vi "View Data.vi"() -> ()   [LabVIEW 2019]
panel:
  in  "X":u16(ring) items=["F1:TIME", "F1:T-TYPE TC #1", "F1:", "F1:"]
  in  "Data File 4":path
  in  "Data File 3":path
  in  "Data File 2":path
  in  "Data File 1":path
  in  "Display Type":enum16{"Stacked Display", "Combined Display"}(ring)
  in  "Y4":u16(ring) items=["F1:TIME", "F1:T-TYPE TC #1", "F1:", "F1:"]
  in  "Y3":u16(ring) items=["F1:TIME", "F1:T-TYPE TC #1", "F1:", "F1:"]
  in  "Y2":u16(ring) items=["F1:TIME", "F1:T-TYPE TC #1", "F1:", "F1:"]
  in  "Y1":u16(ring) items=["F1:TIME", "F1:T-TYPE TC #1", "F1:", "F1:"]
  out "Graph":cluster{dbl[], dbl[]}[](graph)
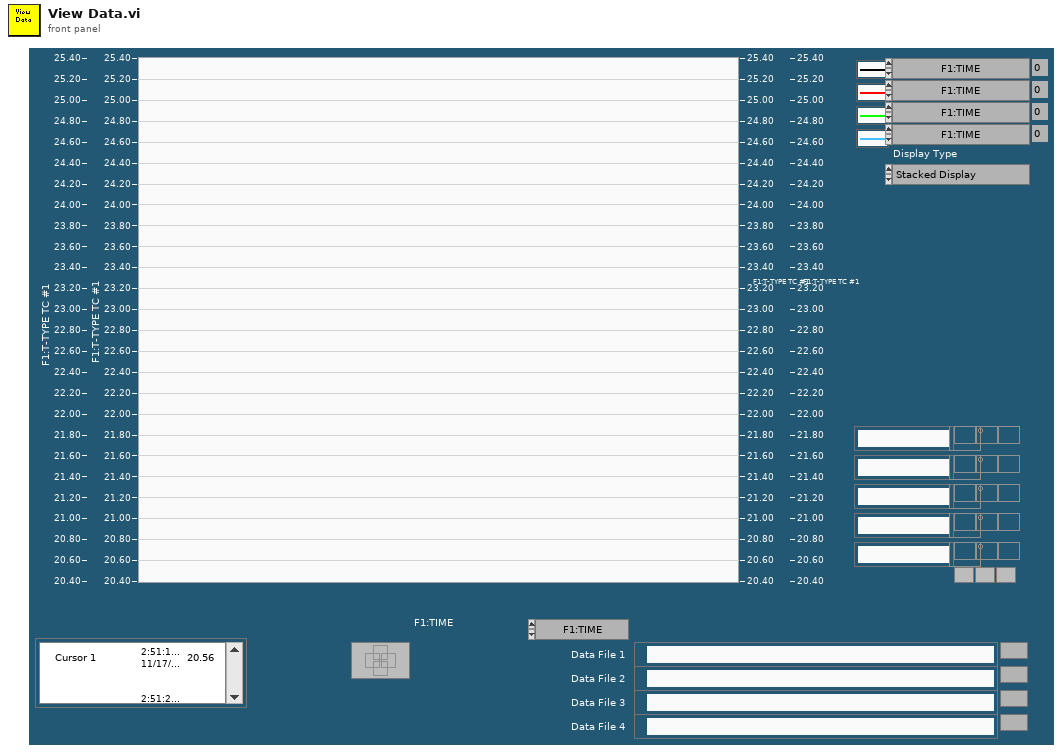
[diagram p1: front panel]
types:
  T1 = cluster{"DAQ Active":bool, "Data File":path, "Index":i32, "Headers":cluster{string[]}[], "Data":cluster{dbl[][]}[], "Sample Rate":dbl[], "Y Axis Names":string[], "X Axis Name":string}
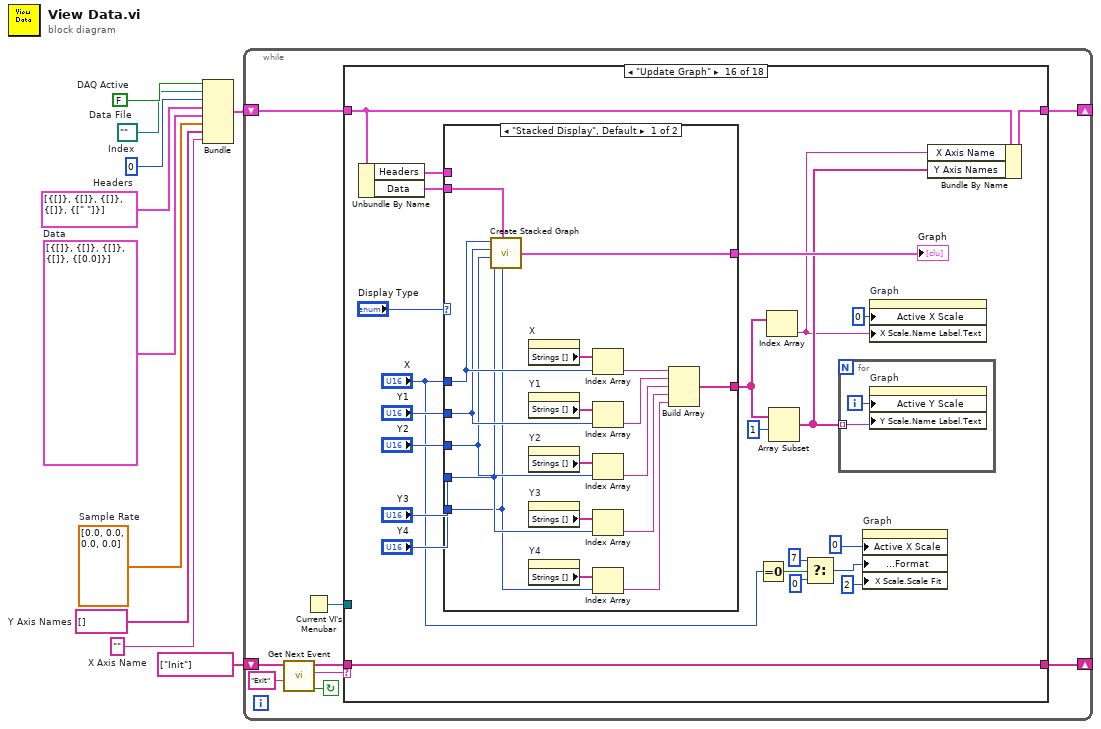
[diagram p0: block diagram]
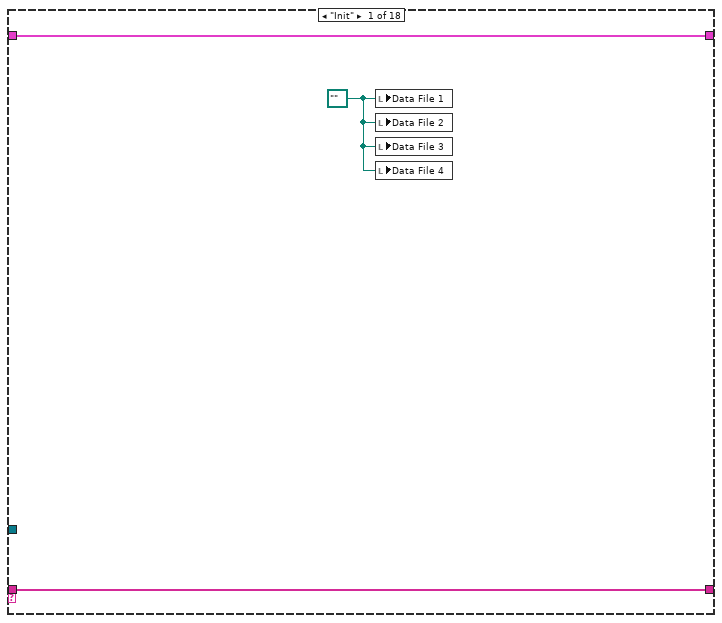
[diagram p2: hidden frame]
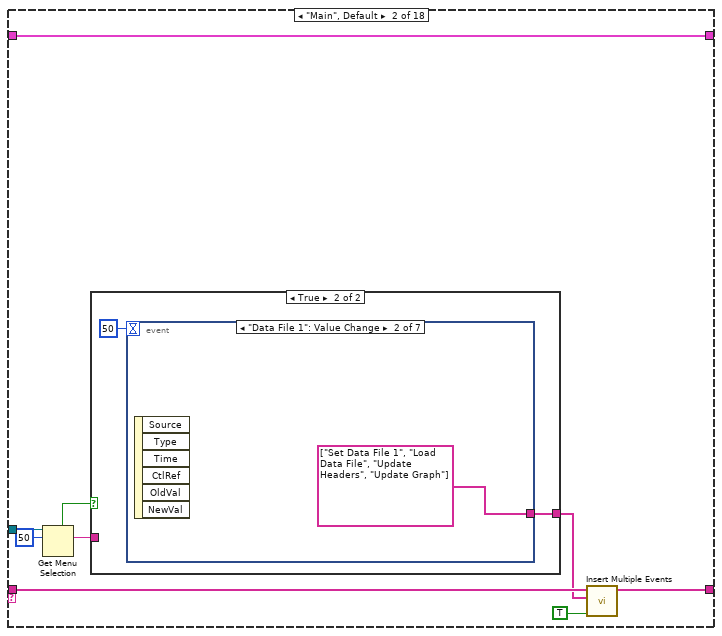
[diagram p3: hidden frame]
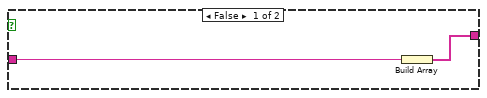
[diagram p4: hidden frame]
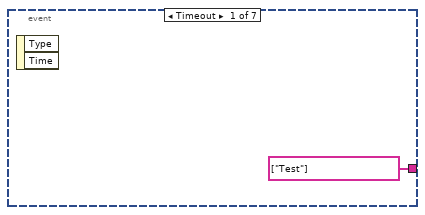
[diagram p5: hidden frame]
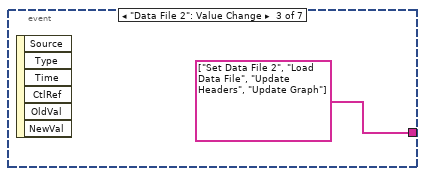
[diagram p6: hidden frame]
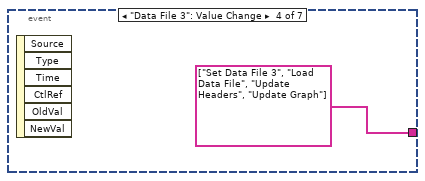
[diagram p7: hidden frame]
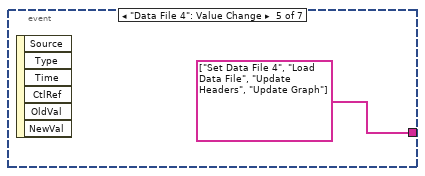
[diagram p8: hidden frame]
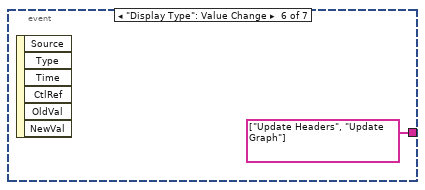
[diagram p9: hidden frame]
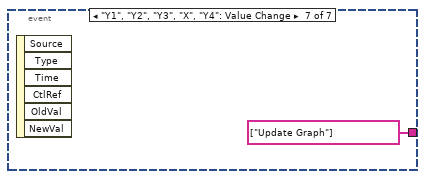
[diagram p10: hidden frame]
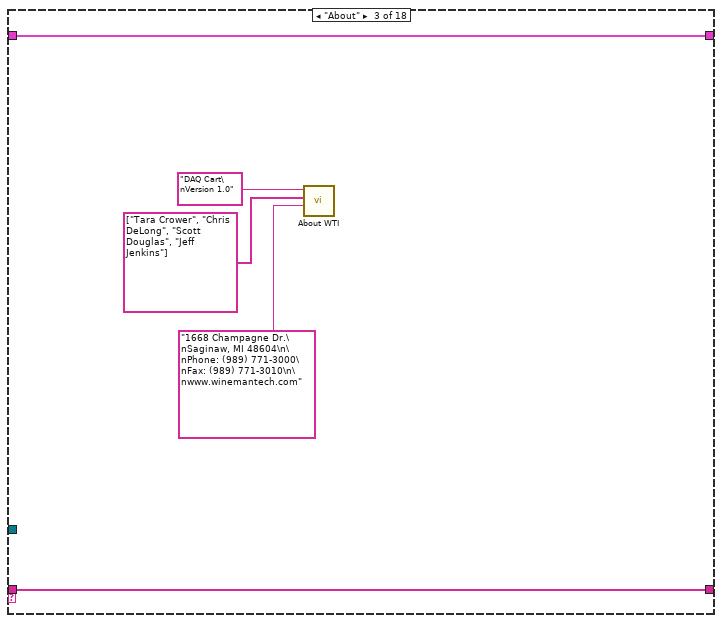
[diagram p11: hidden frame]
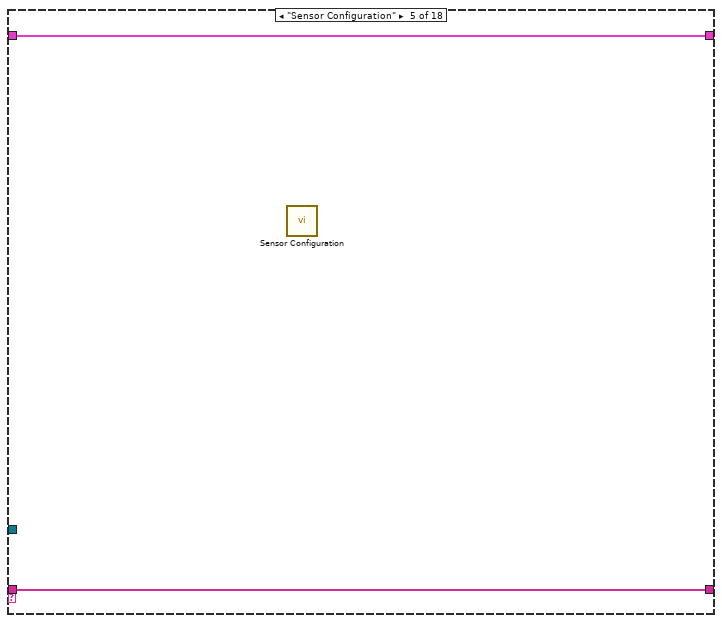
[diagram p13: hidden frame]
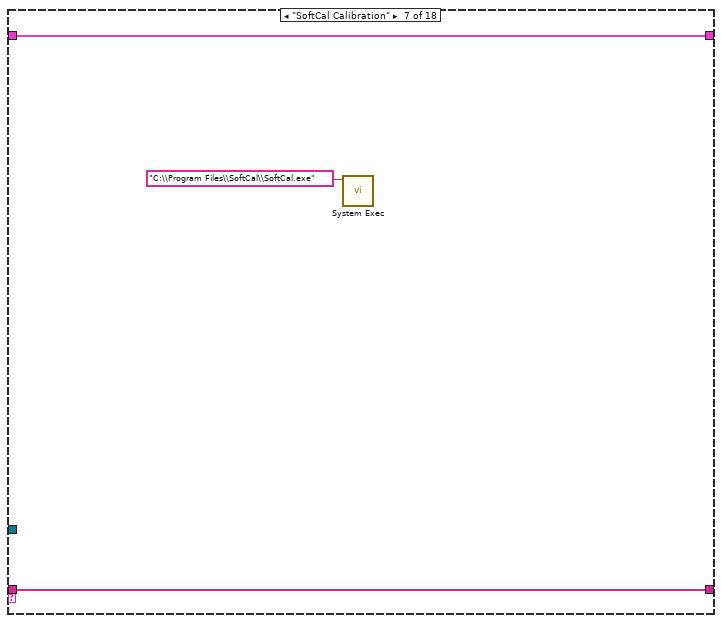
[diagram p15: hidden frame]
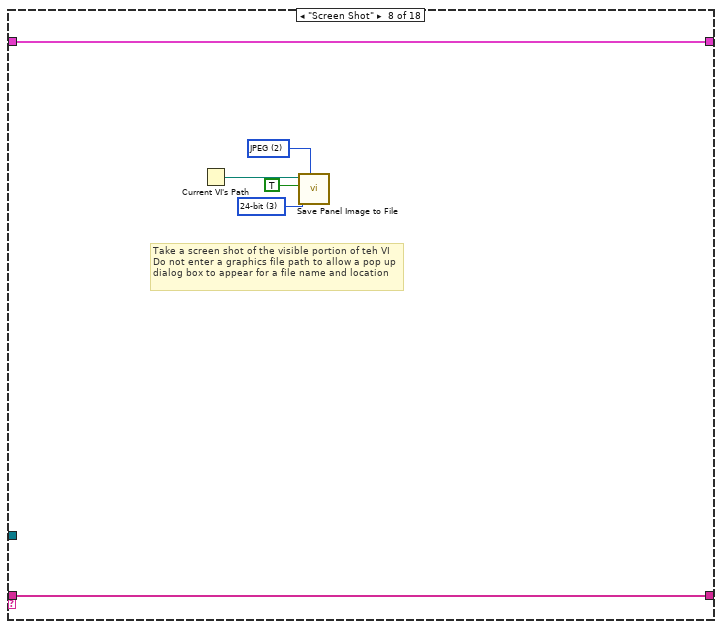
[diagram p16: hidden frame]
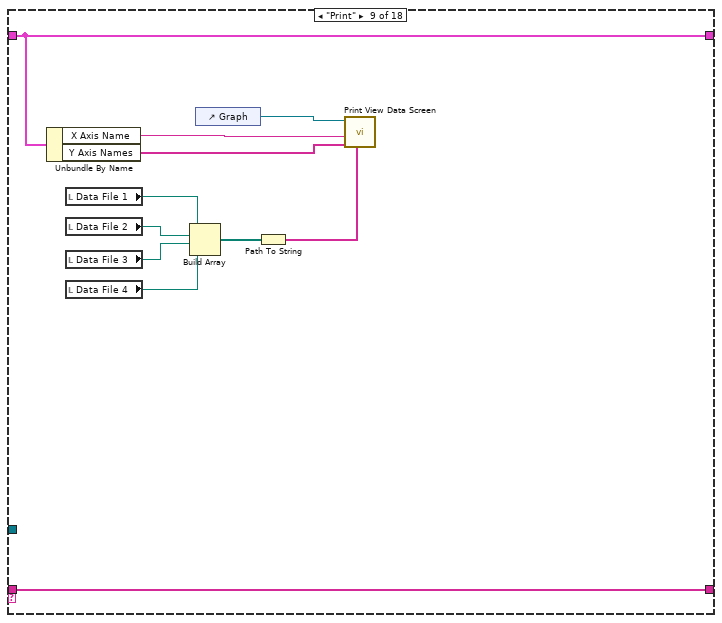
[diagram p17: hidden frame]
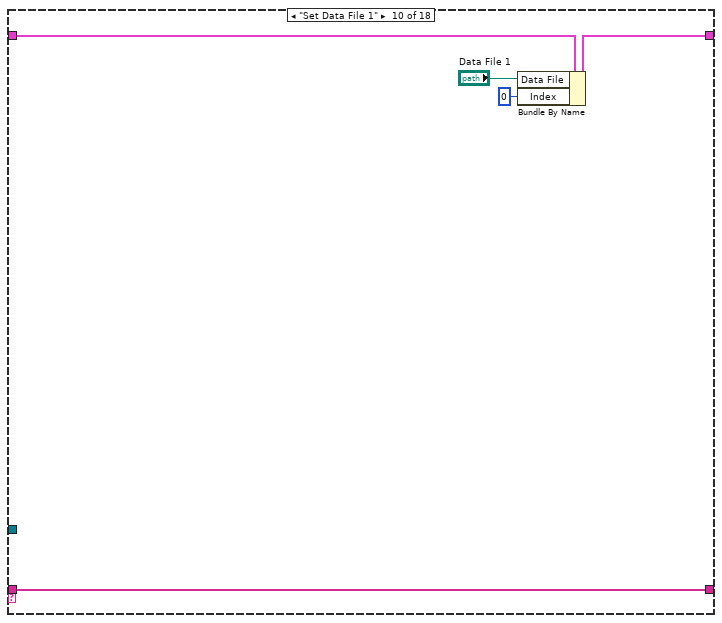
[diagram p18: hidden frame]
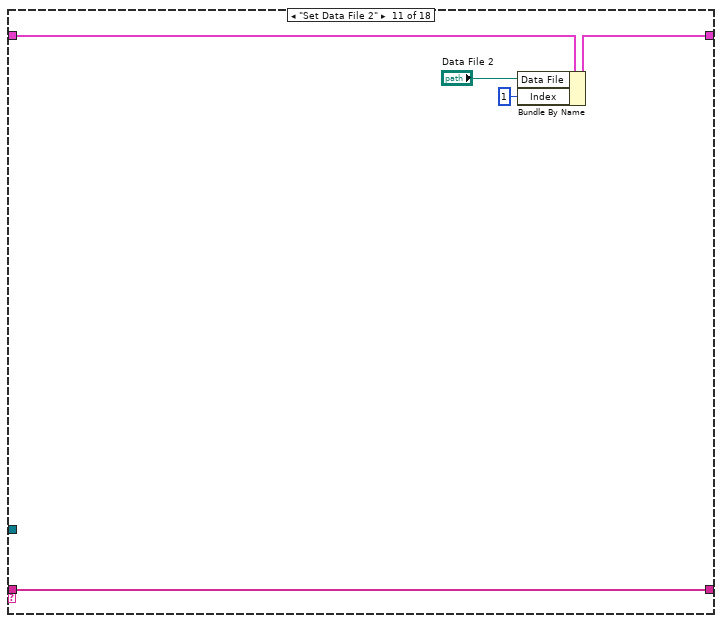
[diagram p19: hidden frame]
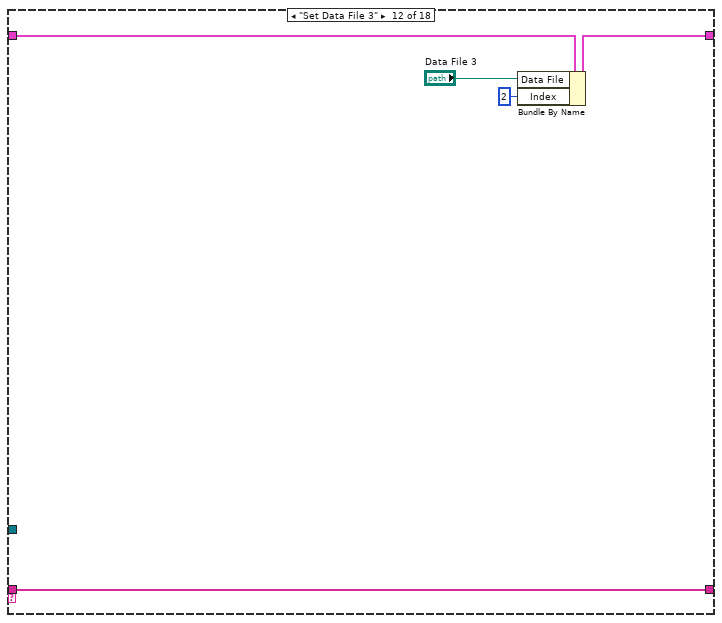
[diagram p20: hidden frame]
diagram:
  w1 = ""  # X Axis Name
  w2 = string[] []  # Y Axis Names
  w3 = dbl[] [0.0, 0.0, 0.0, 0.0]  # Sample Rate
  w6 = 0  # Index
  w4 = cluster{dbl[][]}[] [{[]}, {[]}, {[]}, {[]}, {[[0.0]]}]  # Data
  w5 = cluster{string[]}[] [{[]}, {[]}, {[]}, {[]}, {[" "]}]  # Headers
  w7 = path ""  # Data File
  w8 = FALSE  # DAQ Active
  n1 = Bundle("DAQ Active"=w8, "Data File"=w7, "Index"=w6, "Headers"=w5, "Data"=w4, "Sample Rate"=w3, "Y Axis Names"=w2, "X Axis Name"=w1) -> (w9:T1)  [unwired: 1 in]
  n2 = while {
    shift-left: string[] ["Init"] ("event queue out") -> [w17]
    shift-right: [w14] -> _
    shift-left: w9 -> [w16]
    shift-right: [w11] -> _
    stop <- w19 continue-if-true
    n3 = call "Get Next Event.vi"("Exit Event"="Exit", "event queue in"=w17) -> ("Condition (Exit:F)"=w19:bool, "next event"=w18:string, "event queue out"=w15:string[])  [unwired: 3 in]
    n4 = Current VI's Menubar() -> (w12:refnum<k9>)
    n5 = case shown="\"Update Graph\"" w18 {
      tunnel: w16 -> [w22 w31 w47 w49 w51 w53 w56 w62 w71 w77 w82 w87 w92 w102 w165 w237 w290 w292]
      tunnel: [w21 w30 w46 w48 w50 w52 w55 w61 w73 w78 w83 w88 w93 w103 w173 w246 w289 w291] -> w14
      tunnel: w15 -> [w21 w29 w46 w48 w50 w52 w55 w61 w73 w78 w83 w88 w93 w103 w173 w246 w289 w291]
      tunnel: w12 -> [_ w28 _ _ _ _ _ _ _ _ _ _ _ _ _ _ _ _]
      tunnel: [w22 w31 w47 w49 w51 w53 w56 w62 w71 w76 w81 w86 w91 w101 w165 w236 w290 w292] -> w11
      frame "Init" {
        w20 = path "" ("Data File 1")
        n6 = local write "Data File 1"(w20) -> ()
        n7 = local write "Data File 2"(w20) -> ()
        n8 = local write "Data File 3"(w20) -> ()
        n9 = local write "Data File 4"(w20) -> ()
      }
      frame "Main", Default {
        n10 = Get Menu Selection(0:w28, 1:50 ("ms timeout (200)")) -> (4:w24:bool, 6:w27:string)  [unwired: 2 in, 3 out]
        n11 = case shown="True" w24 {
          tunnel: w27 -> [w33 _]
          tunnel: [w32 w35] -> w26
          frame False {
            n12 = Build Array(w33) -> (w32:string[])
          }
          frame True {
            n13 = event shown="[1] \"Data File 1\": Value Change" {
              selector: _ -> [_ _ _ _ _ _ _]
              dyn-events: _ -> [_ _ _ _ _ _ _]
              timeout: 50 -> [_ _ _ _ _ _ _]
              tunnel: [string[] ["Test"] string[] ["Set Data File 1", "Load Data File", "Update Headers", "Update Graph"] string[] ["Set Data File 2", "Load Data File", "Update Headers", "Update Graph"] string[] ["Set Data File 3", "Load Data File", "Update Headers", "Update Graph"] string[] ["Set Data File 4", "Load Data File", "Update Headers", "Update Graph"] string[] ["Update Headers", "Update Graph"] string[] ["Update Graph"]] -> w35
              event Timeout {
                n14 = event-data() -> ()  [unwired: 1 in, 2 out]
              }
              event "Data File 1": Value Change {
                n15 = event-data() -> ()  [unwired: 1 in, 6 out]
              }
              event "Data File 2": Value Change {
                n16 = event-data() -> ()  [unwired: 1 in, 6 out]
              }
              event "Data File 3": Value Change {
                n17 = event-data() -> ()  [unwired: 1 in, 6 out]
              }
              event "Data File 4": Value Change {
                n18 = event-data() -> ()  [unwired: 1 in, 6 out]
              }
              event "Display Type": Value Change {
                n19 = event-data() -> ()  [unwired: 1 in, 6 out]
              }
              event "Y1", "Y2", "Y3", "X", "Y4": Value Change {
                n20 = event-data() -> ()  [unwired: 1 in, 6 out]
              }
            }
          }
        }
        n21 = call "Insert Multiple Events.vi"("Insert all? (T)"=TRUE, "Events to Insert"=w26, "Event queue in"=w29) -> ("Event queue out"=w30:string[])  [unwired: 4 in]
      }
      frame "About" {
        n22 = call "About WTI.vi"("Description and Version"="DAQ Cart\nVersion 1.0", "Designers"=string[] ["Tara Crower", "Chris DeLong", "Scott Douglas", "Jeff Jenkins"], "Contact Information In"="1668 Champagne Dr.\nSaginaw, MI 48604\n\nPhone: (989) 771-3000\nFax: (989) 771-3010\n\nwww.winemantech.com") -> ()  [unwired: 5 in]
      }
      frame "View Data" {
      }
      frame "Sensor Configuration" {
        n23 = call "Sensor Configuration.vi"() -> ()  [unwired: 15 in, 1 out]
      }
      frame "Simple Calibration" {
      }
      frame "SoftCal Calibration" {
        n24 = call <vilib>:"System Exec.vi"("command line"="C:\\Program Files\\SoftCal\\SoftCal.exe") -> ()  [unwired: 7 in, 4 out]
      }
      frame "Screen Shot" {
        w57 = u16 3 items=["1-bit", "4-bit", "8-bit", "24-bit"] ("Image Depth")
        w60 = u16 2 items=["BMP", "PNG", "JPEG"] ("Graphic File Type")
        # "Take a screen shot of the visible portion of teh VI\nDo not enter a graphics file path to allow a pop up dialog box to appear for a file name and location"
        n25 = Current VI's Path() -> (path=w59:path)
        n26 = call "Save Panel Image to File.vi"("vi path"=w59, "visible area only"=TRUE, "Image Depth"=w57, "Graphic File Type"=w60) -> ()  [unwired: 1 in, 1 out]
      }
      frame "Print" {
        n27 = Unbundle By Name(w71) -> ("X Axis Name"=w70:string, "Y Axis Names"=w69:string[])
        n28 = local read "Data File 1"() -> (w68:path)
        n29 = local read "Data File 2"() -> (w66:path)
        n30 = local read "Data File 3"() -> (w65:path)
        n31 = local read "Data File 4"() -> (w67:path)
        n32 = Build Array(w68, w66, w65, w67) -> (w64:path[])
        n33 = control-ref of="Graph"() -> (w72:refnum<vi>)
        n34 = Path To String(path=w64) -> (string=w63:string[])
        n35 = call "Print View Data Screen.vi"("file names"=w63, "Y Axis Names"=w69, "X Axis Name"=w70, "Graph Ref  in"=w72) -> ()  [unwired: 8 in]
      }
      frame "Set Data File 1" {
        n36 = Bundle By Name(cluster=w77, "Data File"="Data File 1", "Index"=0) -> (w76:T1)
      }
      frame "Set Data File 2" {
        n37 = Bundle By Name(cluster=w82, "Data File"="Data File 2", "Index"=1) -> (w81:T1)
      }
      frame "Set Data File 3" {
        n38 = Bundle By Name(cluster=w87, "Data File"="Data File 3", "Index"=2) -> (w86:T1)
      }
      frame "Set Data File 4" {
        n39 = Bundle By Name(cluster=w92, "Data File"="Data File 4", "Index"=3) -> (w91:T1)
      }
      frame "Load Data File" {
        n40 = Unbundle By Name(w102) -> ("Headers"=w100:cluster{string[]}[], "Data"=w98:cluster{dbl[][]}[], "Index"=w99:i32, "Sample Rate"=w94:dbl[], "Data File"=w95:path)
        n41 = Not Equal?(x=w95, y=path "") -> (x != y?=w97:bool)
        n42 = case shown="True" w97 {
          tunnel: w102 -> [w110 w164]
          tunnel: [w109 w163] -> w101
          tunnel: w95 -> [w108 _]
          tunnel: w100 -> [w107 w162]
          tunnel: w99 -> [w106 w161]
          tunnel: w98 -> [w105 w160]
          tunnel: w94 -> [w104 _]
          frame True {
            n43 = call "Read Characters From File with Error Out.vi"("file path (dialog if empty)"=w108, "[pattern]"="*.csv") -> ("character string"=w111:string, "error out"=w112:errorcluster)  [unwired: 9 in, 3 out]
            n44 = case shown="No Error" w112 {
              tunnel: w111 -> [w152 _]
              tunnel: w110 -> [w150 w153]
              tunnel: [w149 w153] -> w109
              tunnel: w107 -> [w144 _]
              tunnel: w106 -> [w132 _]
              tunnel: w105 -> [w138 _]
              tunnel: w104 -> [w129 _]
              frame No Error {
                # "Row 0 - Time and Date\nRow 1 - Test Description\nRow 2 - Headers\nRow 3... - Data"
                n45 = Spreadsheet String To Array(delimiter (Tab)=",", format string="%s", spreadsheet string=w152, array type (2D Dbl)=string[][] [[""]]) -> (array=w123:string[][])
                n46 = Array Subset(array=w123, index (row)=5 ("index"), index (col)=0 ("index"), length (col)=1 ("index")) -> (w122:string[][])  [unwired: 1 in]
                n47 = Index Array(array=w122, index (col)=0 ("disabled index (col)")) -> (element=w121:string[])  [unwired: 1 in]
                n48 = call "Timestamps to Seconds.vi"("Timestamps"=w121) -> ("Times"=w120:dbl[])  [unwired: 10 in]
                n49 = Index Array(array=w123, index (row)=3) -> (element=w143:string[])  [unwired: 1 in]
                n50 = Array Subset(array=w123, index (row)=5 ("index"), index (col)=1 ("index")) -> (w139:string[][])  [unwired: 2 in]
                n51 = Fract/Exp String To Number(string=w139) -> (number=w119:dbl[][])  [unwired: 3 in, 1 out]
                n52 = Transpose 2D Array(2D array=w119) -> (transposed array=w118:dbl[][])
                n53 = Build Array (concatenate)(w120, w118) -> (w117:dbl[][])
                n54 = Transpose 2D Array(2D array=w117) -> (transposed array=w116:dbl[][])
                n55 = Bundle(w143) -> (w142:cluster{string[]})  [unwired: 1 in]
                n56 = Bundle(w116) -> (w137:cluster{dbl[][]})  [unwired: 1 in]
                n57 = Replace Array Subset(array=w144, new element=w142, index=w132) -> (w148:cluster{string[]}[])
                n58 = Replace Array Subset(array=w138, new element=w137, index=w132) -> (w136:cluster{dbl[][]}[])
                n59 = Index Array(array=w120, index #1=0 ("index (row)"), index #2=1 ("index (row)")) -> (element #1=w128:dbl, element #2=w127:dbl)
                n60 = Subtract(x=w128, y=w127) -> (x-y=w133:dbl)
                n61 = Reciprocal(x=w133) -> (1/x=w131:dbl)
                n62 = Absolute Value(x=w131) -> (abs(x)=w126:dbl)
                n63 = Replace Array Subset(array=w129, new element=w126, index=w132) -> (w130:dbl[])
                n64 = Bundle By Name(cluster=w150, "Headers"=w148, "Data"=w136, "Sample Rate"=w130) -> (w149:T1)
              }
              frame Error {
              }
            }
          }
          frame False {
            n65 = Bundle("subarray"=string[] []) -> (w158:cluster{"subarray":string[]})  [unwired: 1 in]
            n66 = Replace Array Subset(array=w162, new element=w158, index=w161) -> (w159:cluster{string[]}[])
            n67 = Bundle("number"=dbl[][] []) -> (w157:cluster{"number":dbl[][]})  [unwired: 1 in]
            n68 = Replace Array Subset(array=w160, new element=w157, index=w161) -> (w156:cluster{dbl[][]}[])
            n69 = Bundle By Name(cluster=w164, "Headers"=w159, "Data"=w156) -> (w163:T1)
          }
        }
      }
      frame "Update Headers" {
        n70 = local read "Display Type"() -> (w172:enum16{"Stacked Display", "Combined Display"})
        n71 = Unbundle By Name(w165) -> ("Headers"=w171:cluster{string[]}[])
        n72 = case shown="\"Stacked Display\", Default" w172 {
          tunnel: w171 -> [w188 w215]
          tunnel: [w174 w201] -> w170
          tunnel: [w174 w201] -> w169
          tunnel: [w174 w201] -> w168
          tunnel: [w174 w201] -> w167
          tunnel: [w174 w201] -> w166
          frame "Stacked Display", Default {
            n73 = Index Array(array=w188, index #1=0 ("index")) -> (element #1=w186:cluster{string[]}, element #2=w183:cluster{string[]}, element #3=w184:cluster{string[]}, element #4=w185:cluster{string[]})  [unwired: 3 in]
            n74 = Unbundle(w186) -> (w182:string[])
            n75 = Unbundle(w183) -> (w179:string[])
            n76 = Unbundle(w184) -> (w180:string[])
            n77 = Unbundle(w185) -> (w181:string[])
            n78 = for {
              tunnel: w182 -> [w200] mode=indexing
              tunnel: [w198] -> w177 mode=indexing
              n79 = Concatenate Strings("F1:" ("string"), w200) -> (w198:string)
            }
            n80 = for {
              tunnel: w179 -> [w197] mode=indexing
              tunnel: [w195] -> w178 mode=indexing
              n81 = Concatenate Strings("F2:" ("string"), w197) -> (w195:string)
            }
            n82 = for {
              tunnel: w180 -> [w194] mode=indexing
              tunnel: [w192] -> w176 mode=indexing
              n83 = Concatenate Strings("F3:" ("string"), w194) -> (w192:string)
            }
            n84 = for {
              tunnel: w181 -> [w191] mode=indexing
              tunnel: [w189] -> w175 mode=indexing
              n85 = Concatenate Strings("F4:" ("string"), w191) -> (w189:string)
            }
            n86 = Build Array (concatenate)(w177, w178, w176, w175) -> (w174:string[])
          }
          frame "Combined Display" {
            # "Initialize comparison value with\na name that surely won't be used\nfor a sensor."
            # "Combine all channel names and\nsort.  After sorting, remove all\nduplicate channel names."
            n87 = Index Array(array=w215, index #1=0 ("index")) -> (element #1=w213:cluster{string[]}, element #2=w210:cluster{string[]}, element #3=w211:cluster{string[]}, element #4=w212:cluster{string[]})  [unwired: 3 in]
            n88 = Unbundle(w213) -> (w209:string[])
            n89 = Unbundle(w210) -> (w208:string[])
            n90 = Unbundle(w211) -> (w207:string[])
            n91 = Unbundle(w212) -> (w206:string[])
            n92 = Build Array (concatenate)(w209, w208, w207, w206) -> (w205:string[])
            n93 = Sort 1D Array(array=w205) -> (sorted array=w203:string[])
            n94 = for {
              tunnel: w203 -> [w219] mode=indexing
              shift-right: [w217] -> _
              shift-left: "12345678987654321---" -> [w216]
              shift-right: [w220] -> w201
              shift-left: string[] [] ("sorted array") -> [w218]
              # "Remove duplicate names"
              n95 = Not Equal?(x=w216, y=w219) -> (x != y?=w221:bool)
              n96 = case shown="True" w221 {
                tunnel: [w223 w226] -> w220
                tunnel: w219 -> [_ w224]
                tunnel: w218 -> [w223 w225]
                tunnel: [w222 w224] -> w217
                tunnel: w216 -> [w222 _]
                frame False {
                }
                frame True {
                  n97 = Build Array (concatenate)(w225, w224) -> (w226:string[])
                }
              }
            }
          }
        }
        n98 = property on="Y1" class="Ring (strict)"("Strings []"=w170) -> ()  [unwired: 2 in, 2 out]
        n99 = property on="Y2" class="Ring (strict)"("Strings []"=w169) -> ()  [unwired: 2 in, 2 out]
        n100 = property on="Y3" class="Ring (strict)"("Strings []"=w168) -> ()  [unwired: 2 in, 2 out]
        n101 = property on="Y4" class="Ring (strict)"("Strings []"=w167) -> ()  [unwired: 2 in, 2 out]
        n102 = property on="X" class="Ring (strict)"("Strings []"=w166) -> ()  [unwired: 2 in, 2 out]
      }
      frame "Update Graph" {
        n103 = Unbundle By Name(w237) -> ("Headers"=w241:cluster{string[]}[], "Data"=w248:cluster{dbl[][]}[])
        n104 = case shown="\"Stacked Display\", Default" "Display Type" {
          tunnel: w248 -> [w269 w286]
          tunnel: [w268 w288] -> w247
          tunnel: "X" -> [w260 w280]
          tunnel: "Y1" -> [w259 w279]
          tunnel: "Y2" -> [w255 w278]
          tunnel: "Y3" -> [w254 w277]
          tunnel: "Y4" -> [w253 w276]
          tunnel: w241 -> [_ w287]
          tunnel: [w252 w270] -> w240
          frame "Stacked Display", Default {
            n105 = call "Create Stacked Graph.vi"("Y4"=w253, "Data"=w269, "Y3"=w254, "Y2"=w255, "Y1"=w259, "X"=w260) -> ("Graph"=w268:cluster{dbl[], dbl[]}[])
            n106 = property on="X" class="Ring (strict)"() -> ("Strings []"=w256:string[])  [unwired: 2 in, 2 out]
            n107 = property on="Y1" class="Ring (strict)"() -> ("Strings []"=w257:string[])  [unwired: 2 in, 2 out]
            n108 = property on="Y2" class="Ring (strict)"() -> ("Strings []"=w258:string[])  [unwired: 2 in, 2 out]
            n109 = property on="Y3" class="Ring (strict)"() -> ("Strings []"=w267:string[])  [unwired: 2 in, 2 out]
            n110 = property on="Y4" class="Ring (strict)"() -> ("Strings []"=w266:string[])  [unwired: 2 in, 2 out]
            n111 = Index Array(array=w256, index=w260) -> (element=w265:string)
            n112 = Index Array(array=w257, index=w259) -> (element=w264:string)
            n113 = Index Array(array=w258, index=w255) -> (element=w263:string)
            n114 = Index Array(array=w267, index=w254) -> (element=w262:string)
            n115 = Index Array(array=w266, index=w253) -> (element=w261:string)
            n116 = Build Array(w265, w264, w263, w262, w261) -> (w252:string[])
          }
          frame "Combined Display" {
            n117 = property on="X" class="Ring (strict)"() -> ("Strings []"=w285:string[])  [unwired: 2 in, 2 out]
            n118 = property on="Y1" class="Ring (strict)"() -> ("Strings []"=w284:string[])  [unwired: 2 in, 2 out]
            n119 = property on="Y2" class="Ring (strict)"() -> ("Strings []"=w283:string[])  [unwired: 2 in, 2 out]
            n120 = property on="Y3" class="Ring (strict)"() -> ("Strings []"=w282:string[])  [unwired: 2 in, 2 out]
            n121 = property on="Y4" class="Ring (strict)"() -> ("Strings []"=w281:string[])  [unwired: 2 in, 2 out]
            n122 = Index Array(array=w285, index=w280) -> (element=w275:string)
            n123 = Index Array(array=w284, index=w279) -> (element=w274:string)
            n124 = Index Array(array=w283, index=w278) -> (element=w273:string)
            n125 = Index Array(array=w283) -> ()  [unwired: 1 in, 1 out]
            n126 = Index Array(array=w282, index=w277) -> (element=w272:string)
            n127 = Index Array(array=w281, index=w276) -> (element=w271:string)
            n128 = Build Array(w275, w274, w273, w272, w271) -> (w270:string[])
            n129 = call "Create Combined Graph.vi"("Headers"=w287, "Data"=w286, "Axis Select Array"=w270) -> ("Graph"=w288:cluster{dbl[], dbl[]}[])  [unwired: 12 in]
          }
        }
        "Graph" <- w247
        n130 = Equal To 0?(x="X") -> (x = 0?=w231:bool)
        n131 = Index Array(array=w240) -> (element=w234:string)  [unwired: 1 in]
        n132 = Array Subset(array=w240, index=1) -> (w235:string[])  [unwired: 1 in]
        n133 = Select(t=u8 7 ("X Scale.Format & Precision:Format"), s=w231, f=u8 0 ("X Scale.Format & Precision:Format")) -> (s? t:f=w227:u8)
        n134 = for {
          tunnel: w235 -> [w250] mode=indexing
          i -> [w251]
          n135 = property on="Graph" class="XYGraph (strict)"("Active Y Scale"=w251, "Y Scale.Name Label.Text"=w250) -> ()  [unwired: 2 in, 2 out]
        }
        n136 = property on="Graph" class="XYGraph (strict)"("Active X Scale"=0, "X Scale.Display Format:Format"=w227, "X Scale.Scale Fit"=u8 2) -> ()  [unwired: 2 in, 2 out]
        n137 = property on="Graph" class="XYGraph (strict)"("Active X Scale"=0, "X Scale.Name Label.Text"=w234) -> ()  [unwired: 2 in, 2 out]
        n138 = Bundle By Name(cluster=w237, "X Axis Name"=w234, "Y Axis Names"=w235) -> (w236:T1)
      }
      frame "Test" {
      }
      frame "Exit" {
      }
    }
  }
